vi "Area.vi"(8 "error in":errorcluster, 11 "Solution Triangle in":refnum<class "Solution Triangle.lvclass">) -> (0 "error out":errorcluster, 2 "Numeric":dbl, 3 "Solution Triangle out":refnum<class "Solution Triangle.lvclass">)   [LabVIEW 2015, in "Solution Triangle.lvclass"]
uses:
  Solution Triangle.lvclass
  Solution Triangle.lvclass/Solution Triangle.ctl
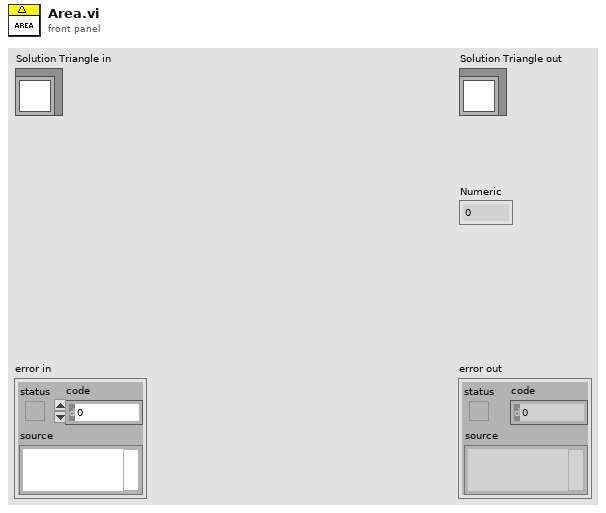
[diagram p1: front panel]
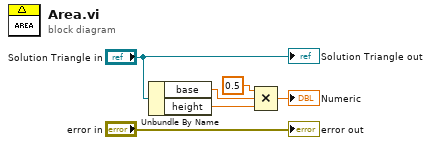
[diagram p0: block diagram]
diagram:
  n1 = Unbundle By Name("Solution Triangle in") -> ("base"=w6:dbl, "height"=w5:dbl)
  n2 = Compound Arithmetic op=MULTIPLY(0.5 ("value"), w6, w5) -> (→"Numeric":dbl)
  "error out" <- "error in"
  "Solution Triangle out" <- "Solution Triangle in"
